vi "AAL Compute H(w) from h(n).vi"(6 "group delay?":bool, 8 "wrap phase?":bool=TRUE, 9 "dB on?":bool=TRUE, 10 "number of frequicies":i32=4096, 11 "h[n]":dbl[](array[numeric]) format="%.2f") -> (1 "df":dbl format="%.2f", 2 "phase":dbl[](array[numeric]) format="%.2f", 3 "amplitude":dbl[](array[numeric]) format="%.2f")   [LabVIEW 2010, in "NI_AALPro.lvlib"]
uses:
  NI_AALPro.lvlib
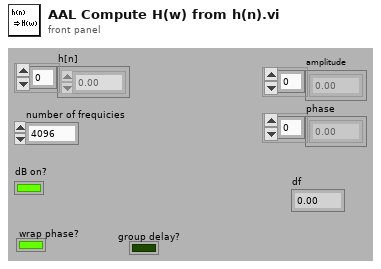
[diagram p1: front panel]
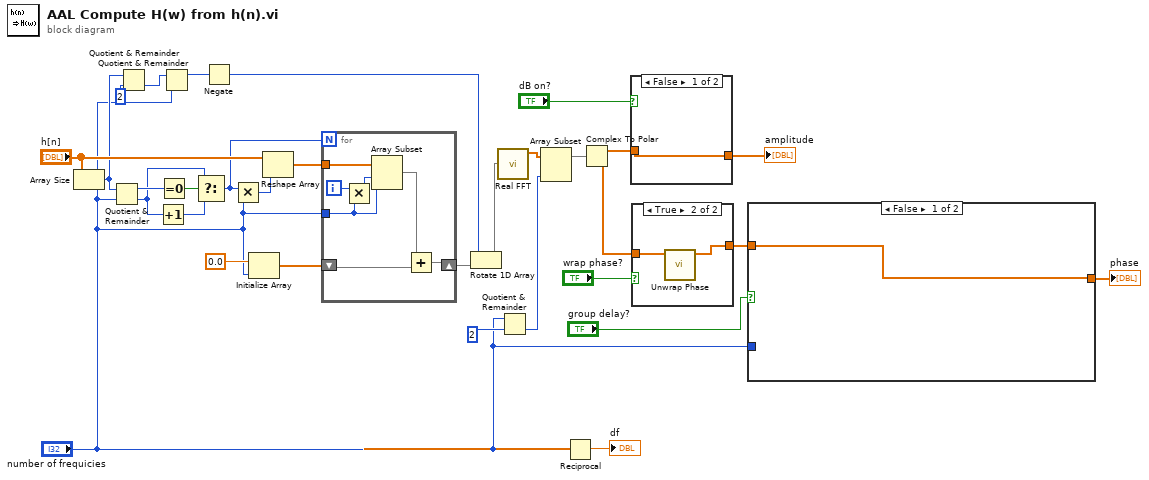
[diagram p0: block diagram]
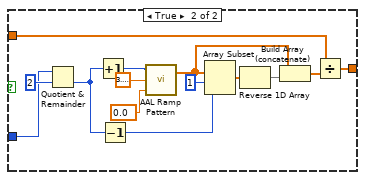
[diagram p2: hidden frame]
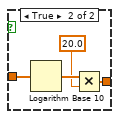
[diagram p4: hidden frame]
diagram:
  n1 = Array Size(array="h[n]") -> (size(s)=w8:i32)
  n2 = Quotient & Remainder(x=w8, y="number of frequicies") -> (x-y*floor(x/y)=w20:i32, floor(x/y)=w17:i32)
  n3 = Quotient & Remainder(x=w8, y=2) -> (floor(x/y)=w2:i32)  [unwired: 1 out]
  n4 = Increment(x=w17) -> (x+1=w18:i32)
  n5 = Equal To 0?(x=w20) -> (x = 0?=w19:bool)
  n6 = Quotient & Remainder(x=w2, y="number of frequicies") -> (x-y*floor(x/y)=w3:i32)  [unwired: 1 out]
  n7 = Select(t=w17, s=w19, f=w18) -> (s? t:f=w13:i32)
  n8 = Negate(x=w3) -> (-x=w1:i32)
  n9 = Multiply(x=w13, y="number of frequicies") -> (x*y=w16:i32)
  n10 = Initialize Array(0.0, "number of frequicies") -> (w15:dbl[])
  n11 = Reshape Array("h[n]", w16) -> (w14:dbl[])
  n12 = for {
    N: w13 -> [_]
    shift-right: [w32] -> w4
    shift-left: w15 -> [w33]
    tunnel: w14 -> [w38]
    tunnel: "number of frequicies" -> [w36]
    i -> [w35]
    n13 = Multiply(x=w35, y=w36) -> (x*y=w37:i32)
    n14 = Array Subset(array=w38, index=w37, length=w36) -> (w34:dbl[])
    n15 = Add(x=w34, y=w33) -> (x+y=w32:dbl[])
  }
  n16 = Rotate 1D Array(1:w4, 2:w1) -> (0:w5:dbl[])
  n17 = call "Real FFT.vi"("X"=w5) -> ("FFT {X}"=w12:cdb[])  [unwired: 9 in, 1 out]
  n18 = Quotient & Remainder(x="number of frequicies", y=2) -> (floor(x/y)=w9:i32)  [unwired: 1 out]
  n19 = Array Subset(array=w12, length=w9) -> (w11:cdb[])  [unwired: 1 in]
  n20 = Reciprocal(x="number of frequicies") -> (1/x=→"df":dbl)
  n21 = Complex To Polar(r * e^(i*theta)=w11) -> (r=w28:dbl[], theta=w31:dbl[])
  n22 = case shown="False" "dB on?" {
    tunnel: w28 -> [w39 w43]
    tunnel: [w39 w41] -> w27
    frame False {
    }
    frame True {
      n23 = Logarithm Base 10(1:w43) -> (0:w42:dbl[])
      n24 = Multiply(x=w42, y=20.0) -> (x*y=w41:dbl[])
    }
  }
  "amplitude" <- w27
  n25 = case shown="True" "wrap phase?" {
    tunnel: w31 -> [w44 w46]
    tunnel: [w44 w45] -> w25
    frame False {
    }
    frame True {
      n26 = call "Unwrap Phase.vi"("Phase"=w46) -> ("Unwrapped Phase"=w45:dbl[])  [unwired: 9 in, 1 out]
    }
  }
  n27 = case shown="False" "group delay?" {
    tunnel: w25 -> [w47 w49]
    tunnel: "number of frequicies" -> [_ w51]
    tunnel: [w47 w48] -> w24
    frame False {
    }
    frame True {
      n28 = Quotient & Remainder(x=w51, y=2) -> (floor(x/y)=w56:i32)  [unwired: 1 out]
      n29 = Increment(x=w56) -> (x+1=w60:i32)
      n30 = Decrement(x=w56) -> (x-1=w55:i32)
      n31 = call "AAL Ramp Pattern.vi"("start"=0.0, "end"=3.141592653589793, "samples"=w60) -> ("Ramp Pattern"=w52:dbl[])  [unwired: 1 out]
      n32 = Array Subset(array=w52, index=1 ("Array Index"), length=w55) -> (w54:dbl[])
      n33 = Reverse 1D Array(array=w54) -> (reversed array=w53:dbl[])
      n34 = Build Array (concatenate)(w52, w53) -> (w50:dbl[])
      n35 = Divide(x=w49, y=w50) -> (x/y=w48:dbl[])
    }
  }
  "phase" <- w24
